vi "Refresh Tag Exchange Booleans.vi"(6 "Tag Exchange Tab References":T1, 8 "error in (no error)":errorcluster, 11 "E2E editor node in":refnum<data-value>) -> (0 "error out":errorcluster, 3 "E2E editor node out":refnum<data-value>)   [LabVIEW 2015, in "E2E Tag Exchange editor node.lvclass"]
uses:
  E2E Tag Exchange editor node.lvclass
  Tag Exchange Tab References.ctl
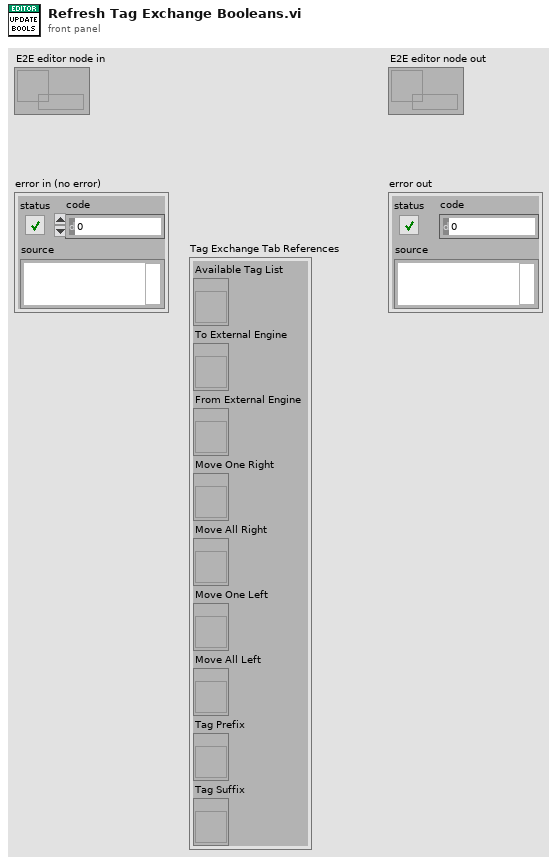
[diagram p1: front panel]
types:
  T1 = typedef "E2E Tag Exchange editor node.lvclass/Tag Exchange Tab References.ctl" = cluster{"Available Tag List":refnum<vi>, "To External Engine":refnum<vi>, "From External Engine":refnum<vi>, "Move One Right":refnum<vi>, "Move All Right":refnum<vi>, "Move One Left":refnum<vi>, "Move All Left":refnum<vi>, "Tag Prefix":refnum<vi>, "Tag Suffix":refnum<vi>}
  T2 = enum8{"Enabled", "Disabled", "Disabled and Grayed Out"}
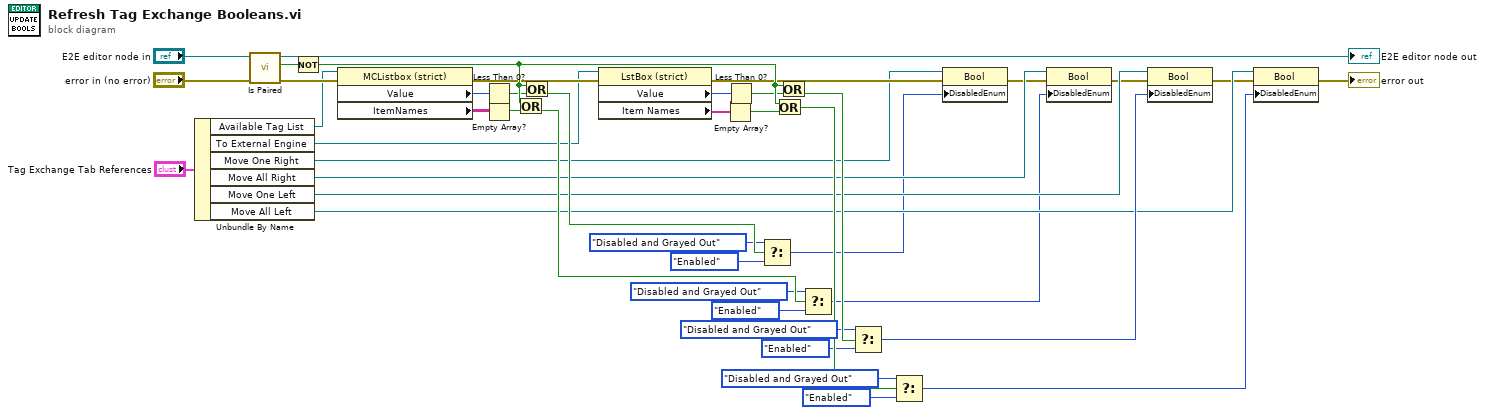
[diagram p0: block diagram]
diagram:
  n1 = Unbundle By Name("Tag Exchange Tab References") -> ("Available Tag List"=w2:refnum<vi>, "To External Engine"=w5:refnum<vi>, "Move One Right"=w7:refnum<vi>, "Move All Right"=w15:refnum<vi>, "Move One Left"=w21:refnum<vi>, "Move All Left"=w22:refnum<vi>)
  n2 = call "Is Paired.vi"("error in (no error)"="error in (no error)", "E2E editor node in"="E2E editor node in") -> ("error out"=w33:errorcluster, "Paired?"=w37:bool, "E2E editor node out"=→"E2E editor node out":refnum<data-value>)  [unwired: 7 in]
  n3 = Not(x=w37) -> (.not. x?=w41:bool)
  n4 = property class="MCListbox (strict)"(reference=w2, error in=w33) -> (error out=w6:errorcluster, "Value"=w3:i32, "ItemNames"=w8:string[][])  [unwired: 1 out]
  n5 = Less Than 0?(x=w3) -> (x < 0?=w34:bool)
  n6 = Empty Array?(array=w8) -> (empty?=w35:bool)
  n7 = Or(x=w41, y=w35) -> (x .or. y?=w38:bool)
  n8 = Or(x=w41, y=w34) -> (x .or. y?=w36:bool)
  n9 = property class="LstBox (strict)"(reference=w5, error in=w6) -> (error out=w10:errorcluster, "Value"=w4:i32, "Item Names"=w9:string[])  [unwired: 1 out]
  n10 = Empty Array?(array=w9) -> (empty?=w30:bool)
  n11 = Less Than 0?(x=w4) -> (x < 0?=w29:bool)
  n12 = Select(t=T2."Disabled and Grayed Out", s=w36, f=T2."Enabled" ("Disabled")) -> (s? t:f=w13:T2)
  n13 = Or(x=w41, y=w30) -> (x .or. y?=w40:bool)
  n14 = Or(x=w41, y=w29) -> (x .or. y?=w39:bool)
  n15 = Select(t=T2."Disabled and Grayed Out", s=w38, f=T2."Enabled" ("Disabled")) -> (s? t:f=w18:T2)
  n16 = Select(t=T2."Disabled and Grayed Out", s=w39, f=T2."Enabled" ("Disabled")) -> (s? t:f=w27:T2)
  n17 = Select(t=T2."Disabled and Grayed Out", s=w40, f=T2."Enabled" ("Disabled")) -> (s? t:f=w28:T2)
  n18 = property class="Bool"(reference=w7, error in=w10, "DisabledEnum"=w13) -> (error out=w14:errorcluster)  [unwired: 1 out]
  n19 = property class="Bool"(reference=w15, error in=w14, "DisabledEnum"=w18) -> (error out=w19:errorcluster)  [unwired: 1 out]
  n20 = property class="Bool"(reference=w21, error in=w19, "DisabledEnum"=w27) -> (error out=w20:errorcluster)  [unwired: 1 out]
  n21 = property class="Bool"(reference=w22, error in=w20, "DisabledEnum"=w28) -> (error out=→"error out":errorcluster)  [unwired: 1 out]
